vi "MEMR-Compute.vi"(0 "State In":T2, 5 "Analysis":T3, 7 "Avg":dbl[][](array[numeric]), 9 "seqIndex":i32) -> (4 "State Out":T2, 8 "freq response":T1)   [LabVIEW 2020]
uses:
  Typedefs/MEMR-Analysis.ctl
  Typedefs/MEMR-Analysis State.ctl
  Utility VIs/Array Manipulation VIs/Irregular Array Subset (DBL).vi
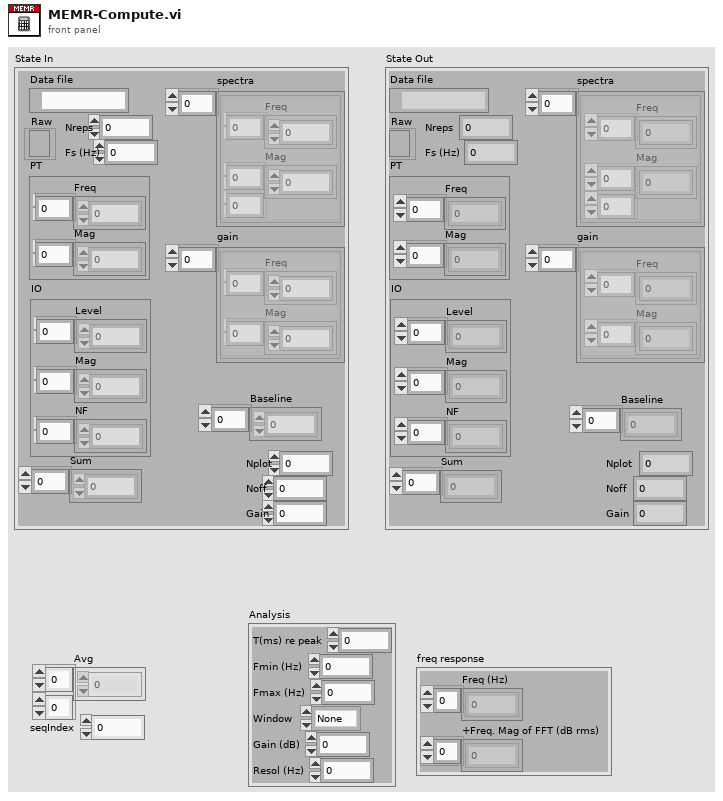
[diagram p1: front panel]
types:
  T1 = cluster{"Freq (Hz)":dbl[], "+Freq. Mag of FFT (dB rms)":dbl[]}
  T2 = typedef "MEMR-Analysis State.ctl" = cluster{"Data file":path, "Raw":refnum<file>, "PT":cluster{"Freq":dbl[], "Mag":dbl[]}, "IO":cluster{"Level":dbl[], "Mag":dbl[], "NF":dbl[]}, "Nreps":i32, "Fs (Hz)":dbl, "Sum":dbl[], "Nplot":i32, "Noff":i32, "Gain":dbl, "spectra":cluster{"Freq":dbl[], "Mag":dbl[][]}[], "gain":cluster{"Freq":dbl[], "Mag":dbl[]}[], "Baseline":dbl[]}
  T3 = typedef "MEMR-Analysis.ctl" = cluster{"T(ms) re peak":dbl, "Fmin (Hz)":dbl, "Fmax (Hz)":dbl, "Window":enum16{"None", "Hanning", "Hamming"}, "Gain (dB)":dbl, "Resol (Hz)":dbl}
  T4 = cluster{"Array Subset":dbl[], "Array Subset":dbl[]}
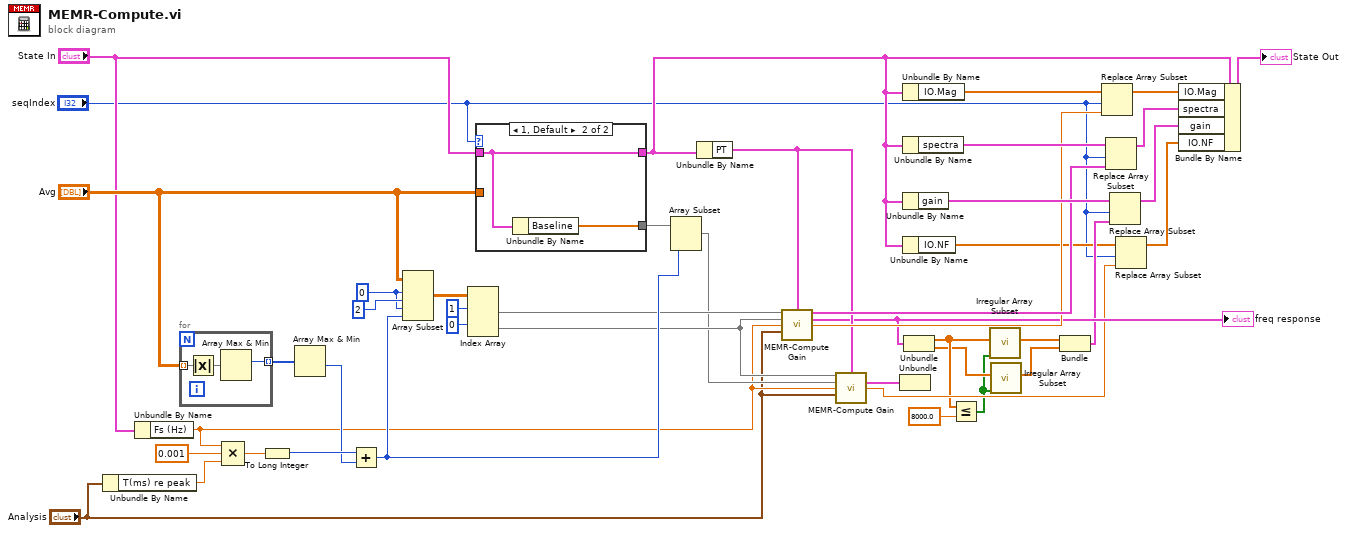
[diagram p0: block diagram]
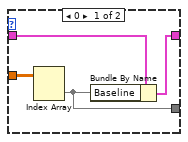
[diagram p2: hidden frame]
diagram:
  w39 = 0 ("index")
  n1 = Unbundle By Name("Analysis") -> ("T(ms) re peak"=w34:dbl)
  n2 = Unbundle By Name("State In") -> ("Fs (Hz)"=w17:dbl)
  n3 = for {
    tunnel: "Avg" -> [w47] mode=indexing
    tunnel: [w46] -> w43 mode=indexing
    n4 = Absolute Value(x=w47) -> (abs(x)=w45:dbl[])
    n5 = Array Max & Min(array=w45) -> (max index (indices)=w46:i32)  [unwired: 3 out]
  }
  n6 = Compound Arithmetic op=MULTIPLY(w17, 0.001 ("value"), w34) -> (w44:dbl)
  n7 = To Long Integer(number=w44) -> (32bit integer=w42:i32)
  n8 = Array Max & Min(array=w43) -> (min value=w41:i32)  [unwired: 3 out]
  n9 = Add(x=w42, y=w41) -> (x+y=w27:i32)
  n10 = Array Subset(array="Avg", index (row)=w39, length (row)=2 ("length"), index (col)=w39, length (col)=w27) -> (w38:dbl[][])
  n11 = Index Array(array=w38, index (row) #1=1 ("index (row)"), index (row) #2=0 ("index (row)")) -> (element #1=w22:dbl[], element #2=w19:dbl[])  [unwired: 2 in]
  n12 = case shown="1, Default" "seqIndex" {
    tunnel: "State In" -> [w50 w52]
    tunnel: [w49 w53] -> w28
    tunnel: "Avg" -> [w51 _]
    tunnel: [w48 w52] -> w10
    frame 0 {
      n13 = Index Array(array=w51) -> (element=w49:dbl[])  [unwired: 2 in]
      n14 = Bundle By Name(cluster=w50, "Baseline"=w49) -> (w48:T2)
    }
    frame 1, Default {
      n15 = Unbundle By Name(w52) -> ("Baseline"=w53:dbl[])
    }
  }
  n16 = Array Subset(array=w28, length=w27) -> (w18:dbl[])  [unwired: 1 in]
  n17 = Unbundle By Name(w10) -> ("PT"=w15:cluster{"Freq":dbl[], "Mag":dbl[]})
  n18 = call "MEMR-Compute Gain.vi"("Test"=w22, "PT"=w15, "Baseline"=w19, "Fs (Hz)"=w17, "Analysis"="Analysis") -> ("spectra"=w21:cluster{"Freq (Hz)":dbl[], dbl[][]}, "gain spectrum"=w14:T1, "Gain (dB)"=w20:dbl)  [unwired: 8 in]
  "freq response" <- w14
  n19 = call "MEMR-Compute Gain.vi"("Test"=w19, "PT"=w15, "Baseline"=w18, "Fs (Hz)"=w17, "Analysis"="Analysis") -> ("gain spectrum"=w13:T1, "Gain (dB)"=w8:dbl)  [unwired: 8 in, 1 out]
  n20 = Unbundle(w13) -> ()  [unwired: 2 out]
  n21 = Unbundle By Name(w10) -> ("IO.Mag"=w33:dbl[])
  n22 = Unbundle By Name(w10) -> ("spectra"=w30:cluster{"Freq":dbl[], "Mag":dbl[][]}[])
  n23 = Unbundle By Name(w10) -> ("gain"=w24:cluster{"Freq":dbl[], "Mag":dbl[]}[])
  n24 = Unbundle By Name(w10) -> ("IO.NF"=w11:dbl[])
  n25 = Unbundle(w14) -> ("Freq (Hz)"=w5:dbl[], "+Freq. Mag of FFT (dB rms)"=w3:dbl[])
  n26 = Less Or Equal?(x=w5, y=8000.0) -> (x <= y?=w1:bool[])
  n27 = call-poly "Irregular Array Subset.vi"("Mask"=w1, "Array"=w5) -> ("Array Subset"=w4:dbl[])  [unwired: 8 in, 1 out]
  n28 = call-poly "Irregular Array Subset.vi"("Mask"=w1, "Array"=w3) -> ("Array Subset"=w2:dbl[])  [unwired: 8 in, 1 out]
  n29 = Bundle("Array Subset"=w4, "Array Subset"=w2) -> (w12:T4)  [unwired: 1 in]
  n30 = Replace Array Subset(array=w33, new element=w20, index="seqIndex") -> (w31:dbl[])
  n31 = Replace Array Subset(array=w30, new element=w21, index="seqIndex") -> (w29:cluster{"Freq":dbl[], "Mag":dbl[][]}[])
  n32 = Replace Array Subset(array=w24, new element=w12, index="seqIndex") -> (w23:cluster{"Freq":dbl[], "Mag":dbl[]}[])
  n33 = Replace Array Subset(array=w11, new element=w8, index="seqIndex") -> (w7:dbl[])
  n34 = Bundle By Name(cluster=w10, "IO.Mag"=w31, "spectra"=w29, "gain"=w23, "IO.NF"=w7) -> (→"State Out":T2)
